vi "Pot Tests.vi"() -> ()   [LabVIEW 2017]
uses:
  <vilib>/FPGAPlugInAG/myRIO-1900/niLvFpga_Open_myRIO-1900.vi
  <vilib>/rvi/interface/common/dynamic/niFpgaDynamicAddResources.vi
  <vilib>/Utility/error.llb/Error Cluster From Error Code.vi
  <vilib>/rvi/errors/niLvFpgaAdjustHostInterfaceError.vi
  <vilib>/FPGAPlugInAG/Dynamic/niLvFpga_Close_Dynamic.vi
  <vilib>/rvi/interface/nirviOpenFPGA/nirviOpenFPGA.xnode
  FPGA Bitfiles/myPAM_FPGATarget_FPGA(POTTEST)_k27VEdd3m1w.lvbitx
  FPGA/FPGA (POT TEST).vi
  <vilib>/rvi/interface/nirviReadWriteControl/nirviReadWriteControl.xnode
  <vilib>/rvi/interface/nirviCloseFPGA/nirviCloseFPGA.xnode
  NiFpgaLv.dll
  <vilib>/rvi/interface/Simulation/niFpgaSimulationCallBeginRW.vi
panel:
  out "POT2_POS":u16
  out "POT1_POS":u16
  in  "Stop Button":bool
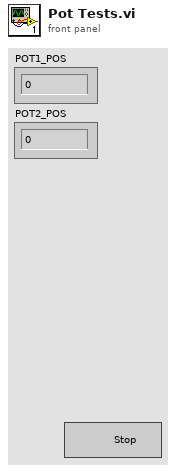
[diagram p1: front panel]
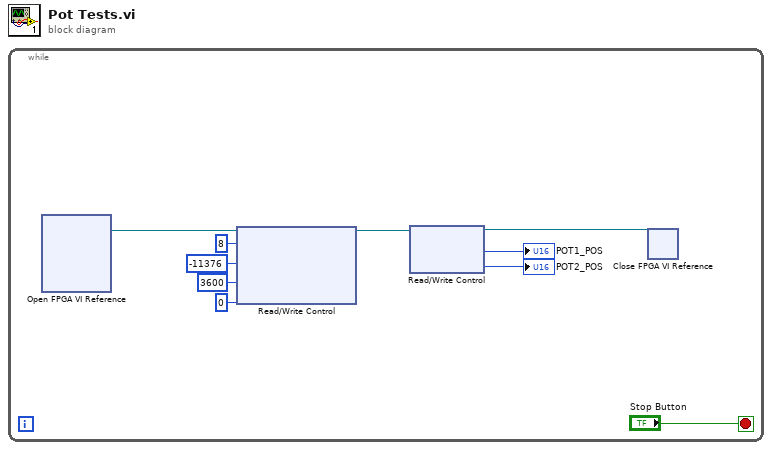
[diagram p0: block diagram]
diagram:
  n1 = while {
    stop <- "Stop Button" stop-if-true
    n2 = xnode "Open FPGA VI Reference"() -> ("FPGA VI Reference Out"=w9:refnum<k20>)  [unwired: 2 in, 1 out]
    n3 = xnode "Read/Write Control"("FPGA VI Reference In"=w9, "LINK1_POT_SCALE"=i16 8, "LINK1_OFFSET"=i16 -11376, "LINK2_POT_SCALE"=i16 3600, "LINK2_OFFSET"=i16 0) -> ("FPGA VI Reference Out"=w8:refnum<k20>)  [unwired: 1 in, 1 out]
    n4 = xnode "Read/Write Control"("FPGA VI Reference In"=w8) -> ("FPGA VI Reference Out"=w7:refnum<k20>, "POT1_POS"=→"POT1_POS":u16, "POT2_POS"=→"POT2_POS":u16)  [unwired: 1 in, 1 out]
    n5 = xnode "Close FPGA VI Reference"("FPGA VI Reference In"=w7) -> ()  [unwired: 1 in, 1 out]
  }
